vi "svx_Timebase Data Changed.vi"(0 "X":dbl[](array[numeric]), 5 "Y":dbl[](array[numeric]), 7 "time reference":dbl[](array[numeric]), 9 "actual samples/rev":dbl=64.0 format="%.2f", 12 "trigger pulse direction":u16(ring)=1 items=["positive going", "negative going"]) -> (4 "probe X data":cluster{"time":dbl[], "amplitude X":dbl[]}, 6 "tacho points X":cluster{dbl[], dbl[]}, 8 "probe Y data":cluster{"time":dbl[], "amplitude Y":dbl[]}, 10 "tacho points Y":cluster{dbl[], dbl[]})   [LabVIEW 2017, in "SVX Timebase.xctl"]
uses:
  <vilib>/addons/_XControls/Timebase Plot/SVX Timebase.xctl
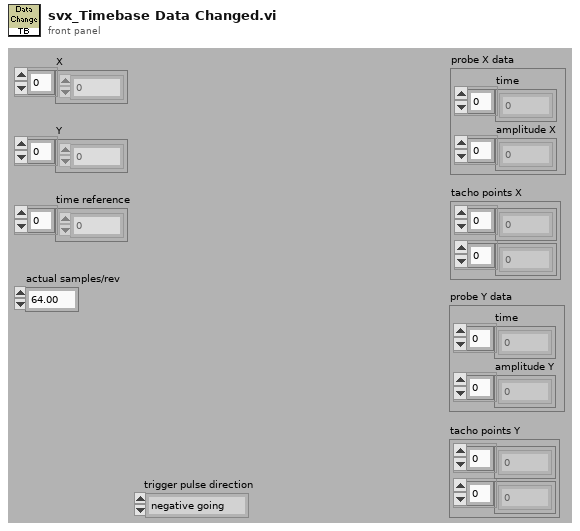
[diagram p1: front panel]
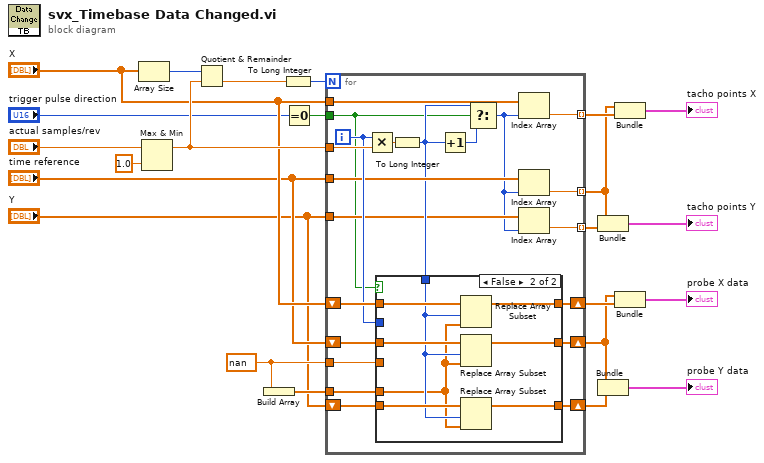
[diagram p0: block diagram]
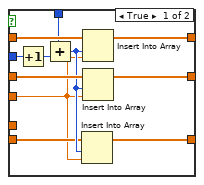
[diagram p2: hidden frame]
diagram:
  w22 = nan ("element")
  n1 = Array Size(array="X") -> (size(s)=w20:i32)
  n2 = Max & Min(x="actual samples/rev", y=1.0) -> (max(x,y)=w15:dbl)  [unwired: 1 out]
  n3 = Quotient & Remainder(x=w20, y=w15) -> (floor(x/y)=w16:dbl)  [unwired: 1 out]
  n4 = Build Array(w22) -> (w21:dbl[])
  n5 = To Long Integer(number=w16) -> (32bit integer=w23:i32)
  n6 = Equal To 0?(x="trigger pulse direction") -> (x = 0?=w1:bool)
  n7 = for {
    N: w23 -> [_]
    tunnel: w15 -> [w41]
    tunnel: [w44] -> w11 mode=indexing
    tunnel: [w43] -> w10 mode=indexing
    tunnel: w21 -> [w40]
    shift-right: [w38] -> w6
    shift-left: "X" -> [w39]
    shift-right: [w37] -> w5
    shift-left: "time reference" -> [w32]
    tunnel: w22 -> [w36]
    tunnel: "X" -> [w34]
    tunnel: "time reference" -> [w33]
    tunnel: "Y" -> [w29]
    tunnel: [w27] -> w9 mode=indexing
    shift-right: [w25] -> w4
    shift-left: "Y" -> [w26]
    tunnel: w1 -> [w24]
    i -> [w35]
    n8 = Multiply(x=w35, y=w41) -> (x*y=w42:dbl)
    n9 = To Long Integer(number=w42) -> (32bit integer=w31:i32)
    n10 = case shown="False" w24 {
      tunnel: w40 -> [_ w57]
      tunnel: w39 -> [w55 w63]
      tunnel: [w50 w62] -> w38
      tunnel: w32 -> [w54 w61]
      tunnel: [w49 w60] -> w37
      tunnel: w31 -> [w53 w58]
      tunnel: w36 -> [w46 _]
      tunnel: w35 -> [w52 _]
      tunnel: w26 -> [w47 w59]
      tunnel: [w45 w56] -> w25
      frame True {
        n11 = Increment(x=w52) -> (x+1=w51:i32)
        n12 = Add(x=w53, y=w51) -> (x+y=w48:i32)
        n13 = Insert Into Array(array=w47, index=w48, new element=w46) -> (w45:dbl[])
        n14 = Insert Into Array(array=w55, index=w48, new element=w46) -> (w50:dbl[])
        n15 = Insert Into Array(array=w54, index=w48, new element=w46) -> (w49:dbl[])
      }
      frame False {
        n16 = Replace Array Subset(array=w63, new element=w57, index=w58) -> (w62:dbl[])
        n17 = Replace Array Subset(array=w61, new element=w57, index=w58) -> (w60:dbl[])
        n18 = Replace Array Subset(array=w59, new element=w57, index=w58) -> (w56:dbl[])
      }
    }
    n19 = Increment(x=w31) -> (x+1=w30:i32)
    n20 = Select(t=w31, s=w24, f=w30) -> (s? t:f=w28:i32)
    n21 = Index Array(array=w34, index=w28) -> (element=w44:dbl)
    n22 = Index Array(array=w33, index=w28) -> (element=w43:dbl)
    n23 = Index Array(array=w29, index=w28) -> (element=w27:dbl)
  }
  n24 = Bundle(w10, w9) -> (→"tacho points Y":cluster{dbl[], dbl[]})  [unwired: 1 in]
  n25 = Bundle("time reference"=w5, "Y"=w4) -> (→"probe Y data":cluster{"time reference":dbl[], "Y":dbl[]})  [unwired: 1 in]
  n26 = Bundle(w10, w11) -> (→"tacho points X":cluster{dbl[], dbl[]})  [unwired: 1 in]
  n27 = Bundle("time reference"=w5, "X"=w6) -> (→"probe X data":cluster{"time reference":dbl[], "X":dbl[]})  [unwired: 1 in]
